vi "svx_SC Line SC Menu.vi"(6 "Run Mode?":bool, 7 "State":T1={"X Scale"={"Name"="Horizontal", "format string"="%#.2g", "Major Color"=16777238, "Minor Color"=16777216, "Scale Visible"=TRUE, " Label Visible"=TRUE, "Grid Style"=1, "Maximum"=1.0, "Minimum"=-1.0}, "Y Scale"={"Name"="Vertical", "format string"="%#.2g", "Major Color"=16777238, "Minor Color"=16777216, "Scale Visible"=TRUE, " Label Visible"=TRUE, "Grid Style"=1, "Maximum"=1.0, "Minimum"=-1.0}, "Plot"={"Point Style"=0, "Line Width"=0, "Line Style"=0, "Plot Color"=16860, "Point/fill"=16860}, "Arrow Color"=16860, "Autoscale"=TRUE, "Property Name"=[], "Container Bounds"={"Width"=550, "Height"=313}, "Background color"=16777226, "Annotation List"=[], "Cursor"={"Cursor Point Style"=13, "Cursor Style"=4, "Cursor Line Width"=1, "Cursor Line Style"=0, "Cursor Color"=16711680, "Cursor Name Visible"=TRUE, "Cursor Visible"=TRUE, "Cursor Position"={"X"=0.0, "Y"=0.0}, "Cursor Index"=0, "Lock Cursor Name"=FALSE, "Cursor reference"=0.0}, "size"=0, "Boundary Color"=9868950, "Maximum"=1.0, "Marker Point Style"=2, "Maker Visible"=TRUE, "Marker Color"=16860, "pair strings []"=[], "clearance boundary"=[{"boundary"={"x axis"=0.0, "y axis"=0.0}, "start point"=enum."center"}], "Custom pair name"=FALSE, "selector.visible"=TRUE, "Cursor Release"=refnum, "Children Tags"=[], "open?"=TRUE, "pair index"=[], "Legend Width"=200, " Parents Tags"="", "Label"="", "Legend Background"=16777226, "Legend Font"=16777222, "scale fit"=2, "user strings []"=[], "Item Width"=0, "out of state queue"=refnum, "property nodes"=refnum, "Kind"=enum."X-Scale", "Scale Range Change"=refnum} {"pair index" min=0; "Y Scale"."Minimum" min=0.0; "Y Scale"."Maximum" min=0.0; "X Scale"."Minimum" min=0.0; "X Scale"."Maximum" min=0.0}, 10 "Refnum":refnum<vi>, 11 "MenuRef":refnum<k9>) -> ()   [LabVIEW 2017, in "SVX SC Line.xctl"]
uses:
  <vilib>/addons/_XControls/Shaft Centerline/SVX SC Line.xctl
  <vilib>/addons/_XControls/Shaft Centerline/subVIs/svx_SC Line State.ctl
  <vilib>/addons/_XControls/Shaft Centerline/subVIs/svx_SC Line Bounds.ctl
  <vilib>/addons/_XControls/Shaft Centerline/subVIs/svx_SC Line Annotation List.ctl
  <vilib>/addons/_XControls/Shaft Centerline/subVIs/svx_SC Line OutState Queue.ctl
panel:
  in  "Run-time\nnew menu":T5(array[cluster])=[{"menu tag"="APP_SC_VISIBLE_ITEMS", "item names"="Plot Legend", "item tags"="USER_SC_SELECTOR", ""}, {"menu tag"="APP_SC_VISIBLE_ITEMS", "item names"="-", "item tags"="APP_SC_SEPERATOR", "USER_SC_SELECTOR"}, {"menu tag"="APP_SC_VISIBLE_ITEMS", "item names"="X Scale", "item tags"="USER_SC_X_SCALE", "APP_SC_SEPERATOR"}, {"menu tag"="APP_SC_VISIBLE_ITEMS", "item names"="Y Scale", "item tags"="USER_SC_Y_SCALE", "USER_SC_X_SCALE"}, {"menu tag"="APP_SC_VISIBLE_ITEMS", "item names"="-", "item tags"="APP_SC_SEPERATOR_2", "USER_SC_Y_SCALE"}, {"menu tag"="APP_SC_VISIBLE_ITEMS", "item names"="Cursor", "item tags"="USER_SC_CURSOR", "APP_SC_SEPERATOR_2"}, {"menu tag"="APP_SC_VISIBLE_ITEMS", "item names"="Cursor Info", "item tags"="USER_SC_CURSORINFO", "USER_SC_CURSOR"}, {"menu tag"="APP_SC_VISIBLE_ITEMS", "item names"="Lock Cursor Info Position", "item tags"="USER_SC_LOCK", "USER_SC_CURSORINFO"}, {"menu tag"="APP_SC_VISIBLE_ITEMS", "item names"="Marker", "item tags"="USER_SC_MARKER", "USER_SC_LOCK"}, {"menu tag"="", "item names"="Autoscale", "item tags"="USER_SC_AUTOSCALE", ""}, {"menu tag"="", "item names"="-", "item tags"="APP_SC_SEPERATOR_3", "USER_SC_AUTOSCALE"}, {"menu tag"="", "item names"="Clearance Boundary", "item tags"="USER_SC_CB", "APP_SC_SEPERATOR_3"}]
  in  "Edit-time\nnew menu":T5(array[cluster])=[{"menu tag"="USER_SC_VISIBLE_ITEMS", "item names"="Label", "item tags"="USER_SC_LABEL", ""}, {"menu tag"="USER_SC_VISIBLE_ITEMS", "item names"="Caption", "item tags"="USER_SC_CAPTION", "USER_SC_LABEL"}, {"menu tag"="USER_SC_VISIBLE_ITEMS", "item names"="-", "item tags"="APP_SC_SEPERATOR", "USER_SC_CAPTION"}, {"menu tag"="USER_SC_VISIBLE_ITEMS", "item names"="Plot Legend", "item tags"="USER_SC_SELECTOR", "APP_SC_SEPERATOR"}, {"menu tag"="USER_SC_VISIBLE_ITEMS", "item names"="-", "item tags"="APP_SC_SEPERATOR_3", "USER_SC_SELECTOR"}, {"menu tag"="USER_SC_VISIBLE_ITEMS", "item names"="X Scale", "item tags"="USER_SC_X_SCALE", "APP_SC_SEPERATOR_3"}, {"menu tag"="USER_SC_VISIBLE_ITEMS", "item names"="Y Scale", "item tags"="USER_SC_Y_SCALE", "USER_SC_X_SCALE"}, {"menu tag"="USER_SC_VISIBLE_ITEMS", "item names"="-", "item tags"="APP_SC_SEPERATOR_4", "USER_SC_Y_SCALE"}, {"menu tag"="USER_SC_VISIBLE_ITEMS", "item names"="Cursor", "item tags"="USER_SC_CURSOR", "APP_SC_SEPERATOR_4"}, {"menu tag"="USER_SC_VISIBLE_ITEMS", "item names"="Cursor Info", "item tags"="USER_SC_CURSORINFO", "USER_SC_CURSOR"}, {"menu tag"="USER_SC_VISIBLE_ITEMS", "item names"="Lock Cursor Info Position", "item tags"="USER_SC_LOCK", "USER_SC_CURSORINFO"}, {"menu tag"="USER_SC_VISIBLE_ITEMS", "item names"="Marker", "item tags"="USER_SC_MARKER", "USER_SC_LOCK"}, {"menu tag"="", "item names"="Autoscale", "item tags"="USER_SC_AUTOSCALE", ""}, {"menu tag"="", "item names"="-", "item tags"="APP_SC_SEPERATOR_2", "USER_SC_AUTOSCALE"}, {"menu tag"="", "item names"="Properties", "item tags"="USER_SC_PROPERTIES", "APP_SC_SEPARATOR_2"}]
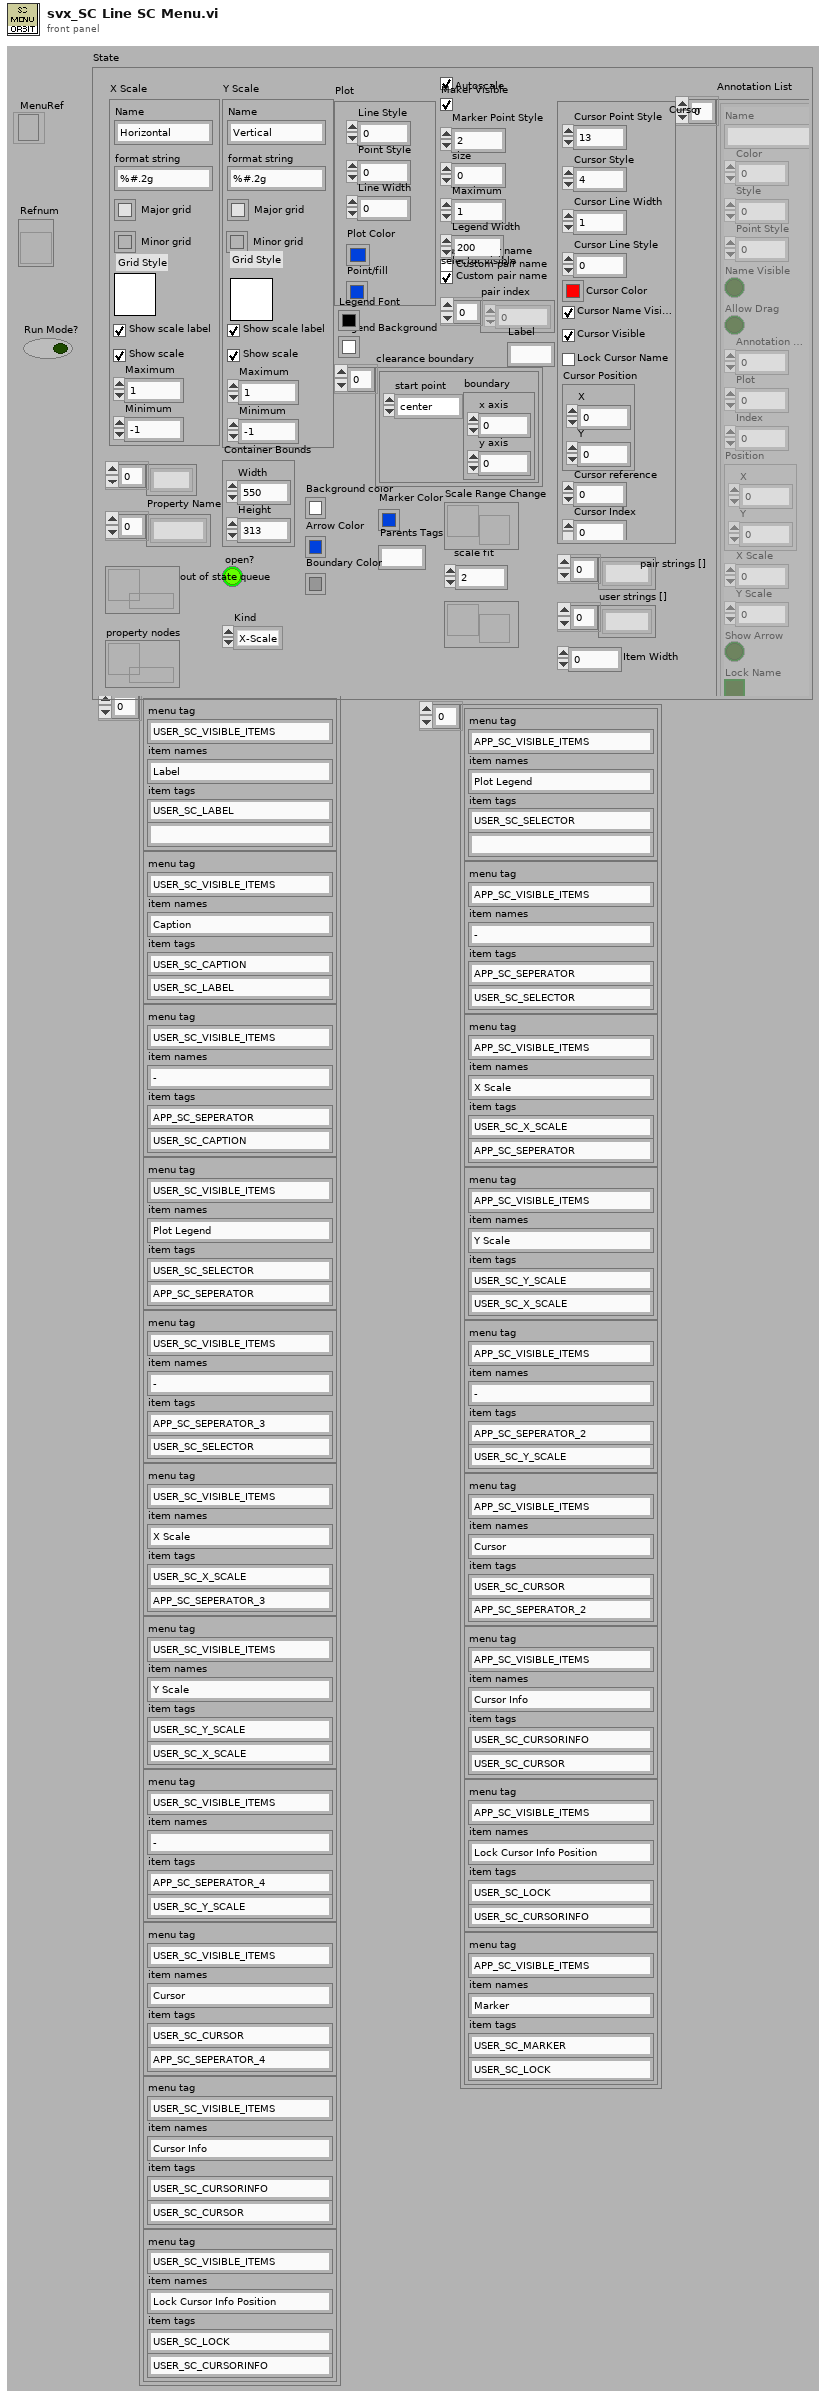
[diagram p1: front panel]
types:
  T1 = typedef "SVX SC Line.xctl/svx_SC Line State.ctl" = cluster{"X Scale":cluster{"Name":string, "format string":string, "Major Color":u32, "Minor Color":u32, "Scale Visible":bool, " Label Visible":bool, "Grid Style":u16, "Maximum":dbl, "Minimum":dbl}, "Y Scale":cluster{"Name":string, "format string":string, "Major Color":u32, "Minor Color":u32, "Scale Visible":bool, " Label Visible":bool, "Grid Style":u16, "Maximum":dbl, "Minimum":dbl}, "Plot":cluster{"Point Style":u8, "Line Width":u8, "Line Style":u8, "Plot Color":u32, "Point/fill":u32}, "Arrow Color":u32, "Autoscale":bool, "Property Name":string[], "Container Bounds":T2, "Background color":u32, "Annotation List":T3, "Cursor":cluster{"Cursor Point Style":u8, "Cursor Style":u8, "Cursor Line Width":u8, "Cursor Line Style":u8, "Cursor Color":u32, "Cursor Name Visible":bool, "Cursor Visible":bool, "Cursor Position":cluster{"X":dbl, "Y":dbl}, "Cursor Index":i32, "Lock Cursor Name":bool, "Cursor reference":dbl}, "size":i32, "Boundary Color":u32, "Maximum":dbl, "Marker Point Style":u8, "Maker Visible":bool, "Marker Color":u32, "pair strings []":string[], "clearance boundary":cluster{"boundary":cluster{"x axis":dbl, "y axis":dbl}, "start point":enum16{"center", "top", "bottom"}}[], "Custom pair name":bool, "selector.visible":bool, "Cursor Release":refnum<user-event>, "Children Tags":string[], "open?":bool, "pair index":i32[], "Legend Width":u32, " Parents Tags":string, "Label":string, "Legend Background":u32, "Legend Font":u32, "scale fit":u8, "user strings []":string[], "Item Width":u32, "out of state queue":T4, "property nodes":refnum<queue>, "Kind":enum16{"X-Scale", "Y-Scale", "Z-Scale"}, "Scale Range Change":refnum<user-event>}
  T2 = typedef "SVX SC Line.xctl/svx_SC Line Bounds.ctl" = cluster{"Width":u32, "Height":u32}
  T3 = typedef "SVX SC Line.xctl/svx_SC Line Annotation List.ctl" = cluster{"Name":string, "Color":u32, "Style":u8, "Point Style":u8, "Name Visible":bool, "Allow Drag":bool, "Annotation Mode":u32, "Plot":i32, "Index":i32, "Position":cluster{"X":dbl, "Y":dbl}, "X Scale":u32, "Y Scale":u32, "Show Arrow":bool, "Lock Name":bool, "Plot Area":i32, "Label Offset":cluster{"X":dbl, "Y":dbl}}[]
  T4 = typedef "SVX SC Line.xctl/svx_SC Line OutState Queue.ctl" = refnum<queue>
  T5 = cluster{"menu tag":string, "item names":string, "item tags":string, string}[]
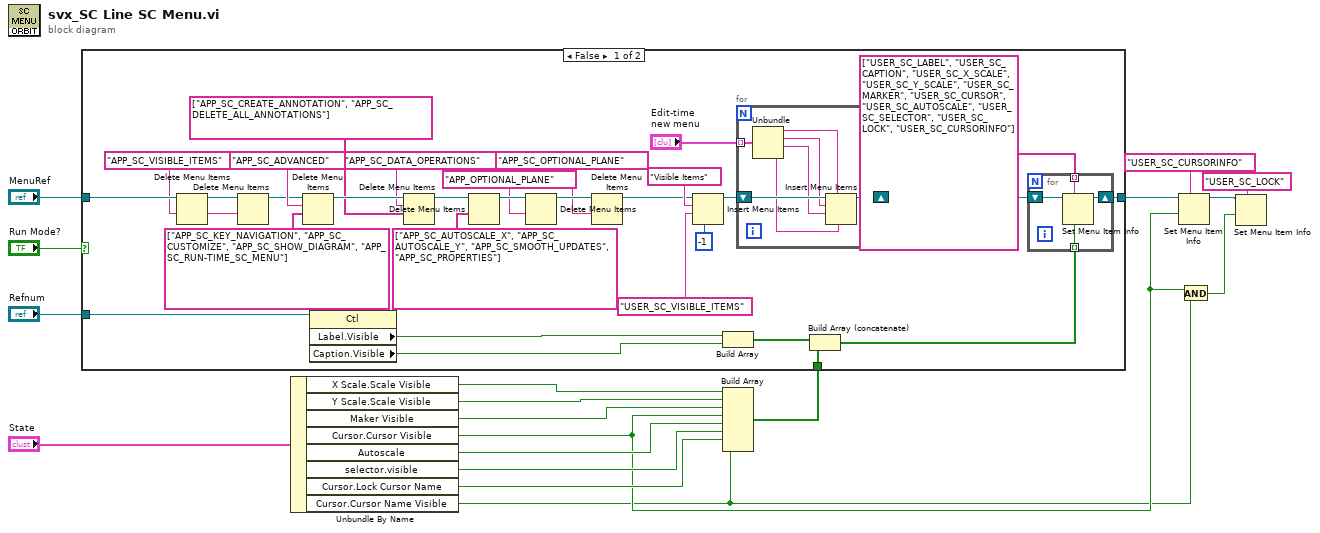
[diagram p0: block diagram]
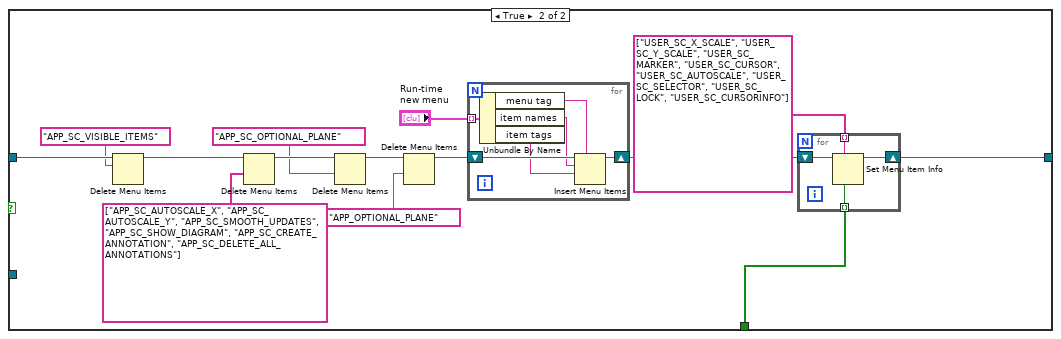
[diagram p2: hidden frame]
diagram:
  n1 = Unbundle By Name("State") -> ("X Scale.Scale Visible"=w15:bool, "Y Scale.Scale Visible"=w14:bool, "Maker Visible"=w10:bool, "Cursor.Cursor Visible"=w3:bool, "Autoscale"=w11:bool, "selector.visible"=w8:bool, "Cursor.Lock Cursor Name"=w9:bool, "Cursor.Cursor Name Visible"=w2:bool)
  n2 = Build Array(w15, w14, w10, w3, w11, w8, w9, w2) -> (w13:bool[])
  n3 = case shown="False" "Run Mode?" {
    tunnel: "MenuRef" -> [w43 w73]
    tunnel: "Refnum" -> [w33 _]
    tunnel: w13 -> [w29 w65]
    tunnel: [w19 w60] -> w7
    frame False {
      w40 = "APP_SC_VISIBLE_ITEMS" ("menu tag")
      n4 = Delete Menu Items(7:w40, 9:w43) -> (3:w42:refnum<k9>)  [unwired: 2 in, 1 out]
      n5 = Delete Menu Items(7:w40, 9:w42) -> (3:w41:refnum<k9>)  [unwired: 2 in, 1 out]
      n6 = Delete Menu Items(7:string[] ["APP_SC_KEY_NAVIGATION", "APP_SC_CUSTOMIZE", "APP_SC_SHOW_DIAGRAM", "APP_SC_RUN-TIME_SC_MENU"], 8:"APP_SC_ADVANCED" ("menu tag"), 9:w41) -> (3:w27:refnum<k9>)  [unwired: 1 in, 1 out]
      n7 = property class="Ctl"(reference=w33) -> ("Label.Visible"=w32:bool, "Caption.Visible"=w31:bool)  [unwired: 1 in, 2 out]
      n8 = Delete Menu Items(7:string[] ["APP_SC_CREATE_ANNOTATION", "APP_SC_DELETE_ALL_ANNOTATIONS"], 8:"APP_SC_DATA_OPERATIONS" ("menu tag"), 9:w27) -> (3:w26:refnum<k9>)  [unwired: 1 in, 1 out]
      n9 = Delete Menu Items(7:string[] ["APP_SC_AUTOSCALE_X", "APP_SC_AUTOSCALE_Y", "APP_SC_SMOOTH_UPDATES", "APP_SC_PROPERTIES"], 9:w26) -> (3:w45:refnum<k9>)  [unwired: 2 in, 1 out]
      n10 = Delete Menu Items(7:"APP_OPTIONAL_PLANE" ("menu tag"), 9:w45) -> (3:w22:refnum<k9>)  [unwired: 2 in, 1 out]
      n11 = Delete Menu Items(7:"APP_SC_OPTIONAL_PLANE" ("menu tag"), 9:w22) -> (3:w21:refnum<k9>)  [unwired: 2 in, 1 out]
      n12 = Insert Menu Items(4:-1, 7:"USER_SC_VISIBLE_ITEMS", 8:"Visible Items" ("item names"), 9:w21) -> (3:w36:refnum<k9>)  [unwired: 2 in, 2 out]
      n13 = Build Array(w32, w31) -> (w30:bool[])
      n14 = for {
        shift-right: [w58] -> w35
        shift-left: w36 -> [w59]
        tunnel: "Edit-time\nnew menu" -> [w57] mode=indexing
        n15 = Unbundle(w57) -> ("menu tag"=w56:string, "item names"=w55:string, "item tags"=w54:string, w53:string)
        n16 = Insert Menu Items(4:w53, 5:w56, 7:w54, 8:w55, 9:w59) -> (3:w58:refnum<k9>)  [unwired: 1 in, 2 out]
      }
      n17 = Build Array (concatenate)(w30, w29) -> (w28:bool[])
      n18 = for {
        shift-right: [w51] -> w19
        shift-left: w35 -> [w52]
        tunnel: string[] ["USER_SC_LABEL", "USER_SC_CAPTION", "USER_SC_X_SCALE", "USER_SC_Y_SCALE", "USER_SC_MARKER", "USER_SC_CURSOR", "USER_SC_AUTOSCALE", "USER_SC_SELECTOR", "USER_SC_LOCK", "USER_SC_CURSORINFO"] ("item tags") -> [w50] mode=indexing
        tunnel: w28 -> [w49] mode=indexing
        n19 = Set Menu Item Info(6:w49, 7:w50, 11:w52) -> (3:w51:refnum<k9>)  [unwired: 4 in, 1 out]
      }
    }
    frame True {
      n20 = Delete Menu Items(8:"APP_SC_VISIBLE_ITEMS" ("menu tag"), 9:w73) -> (3:w72:refnum<k9>)  [unwired: 2 in, 1 out]
      n21 = Delete Menu Items(7:string[] ["APP_SC_AUTOSCALE_X", "APP_SC_AUTOSCALE_Y", "APP_SC_SMOOTH_UPDATES", "APP_SC_SHOW_DIAGRAM", "APP_SC_CREATE_ANNOTATION", "APP_SC_DELETE_ALL_ANNOTATIONS"], 9:w72) -> (3:w64:refnum<k9>)  [unwired: 2 in, 1 out]
      n22 = Delete Menu Items(7:"APP_SC_OPTIONAL_PLANE" ("menu tag"), 9:w64) -> (3:w63:refnum<k9>)  [unwired: 2 in, 1 out]
      n23 = Delete Menu Items(7:"APP_OPTIONAL_PLANE" ("menu tag"), 9:w63) -> (3:w70:refnum<k9>)  [unwired: 2 in, 1 out]
      n24 = for {
        tunnel: "Run-time\nnew menu" -> [w82] mode=indexing
        shift-right: [w78] -> w66
        shift-left: w70 -> [w83]
        n25 = Unbundle By Name(w82) -> ("menu tag"=w81:string, "item names"=w80:string, "item tags"=w79:string)
        n26 = Insert Menu Items(5:w81, 7:w79, 8:w80, 9:w83) -> (3:w78:refnum<k9>)  [unwired: 2 in, 2 out]
      }
      n27 = for {
        shift-right: [w76] -> w60
        shift-left: w66 -> [w77]
        tunnel: string[] ["USER_SC_X_SCALE", "USER_SC_Y_SCALE", "USER_SC_MARKER", "USER_SC_CURSOR", "USER_SC_AUTOSCALE", "USER_SC_SELECTOR", "USER_SC_LOCK", "USER_SC_CURSORINFO"] ("item tags") -> [w75] mode=indexing
        tunnel: w65 -> [w74] mode=indexing
        n28 = Set Menu Item Info(6:w74, 7:w75, 11:w77) -> (3:w76:refnum<k9>)  [unwired: 4 in, 1 out]
      }
    }
  }
  n29 = Set Menu Item Info(7:"USER_SC_CURSORINFO" ("String"), 9:w3, 11:w7) -> (3:w6:refnum<k9>)  [unwired: 4 in, 1 out]
  n30 = And(x=w3, y=w2) -> (x .and. y?=w1:bool)
  n31 = Set Menu Item Info(7:"USER_SC_LOCK" ("String"), 9:w1, 11:w6) -> ()  [unwired: 4 in, 2 out]
